vi "ROI entry screen-Arb plane UI setup.vi"(11 "Number of ROI":i32) -> ()   [LabVIEW 2017]
uses:
  Typedefs/ROI ID Enum.ctl
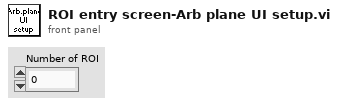
[diagram p1: front panel]
types:
  T1 = typedef "ROI ID Enum.ctl" = enum16{"Point", "MiniScan", "Comp. MiniScan", "Rectangle", "Comp. volume", "Arb. plane point"}
  T2 = enum8{"Enabled", "Disabled", "Disabled and Grayed Out"}
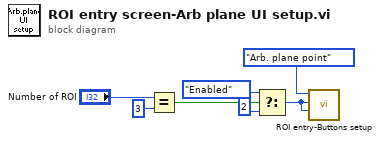
[diagram p0: block diagram]
diagram:
  n1 = Equal?(x="Number of ROI", y=3) -> (x = y?=w4:bool)
  n2 = Select(t=T2."Enabled" ("Disabled"), s=w4, f=2) -> (s? t:f=w3:i32)
  n3 = call "ROI entry-Buttons setup.vi"("Acquisition button disabled?"=w3, "Done button disabled?"=w3, "ROI Enum"=ROI_ID_Enum."Arb. plane point") -> ()  [unwired: 9 in]
